vi "Picture Dial.vi"() -> ()   [LabVIEW 2014]
doc: "Combines a picture control with a dial to have a picture within a dial. The picture control is grouped and locked to the dial along with a decoration to cover the corners of the picture control.\n\n*Notice the use of a stored pixmap image so the image is saved with the VI itself."
uses:
  Rotate.llb/rotate 24bit.vi
panel:
  out "new picture":picture
  in  "Duty Cycle %":dbl(slide)=0.05 scale=0.0..180.0
  in  "stop":bool
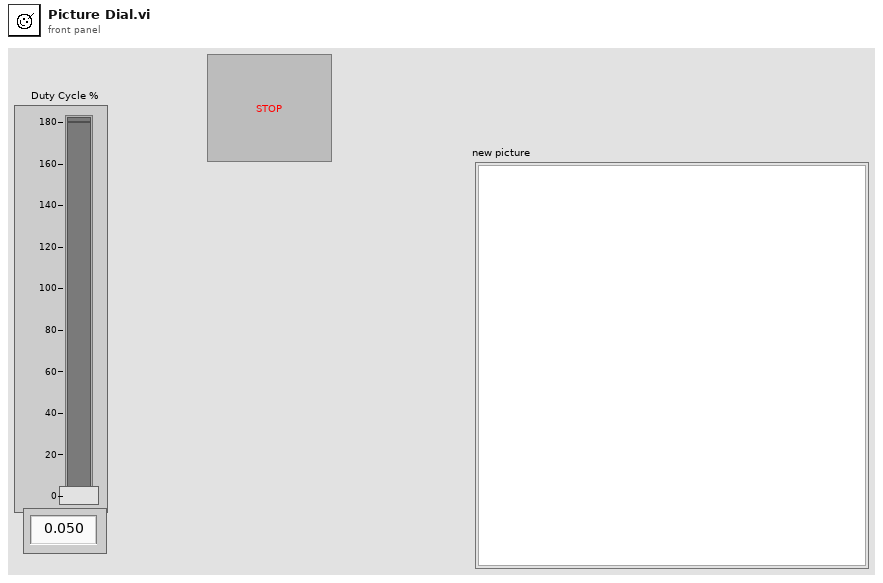
[diagram p1: front panel]
types:
  T1 = typedef "imagedata.ctl" = cluster{"image type":i32, "image depth":i32, "image":u8[], "mask":u8[], "colors":u32[], "Rectangle":cluster{"left":i16, "top":i16, "right":i16, "bottom":i16}}
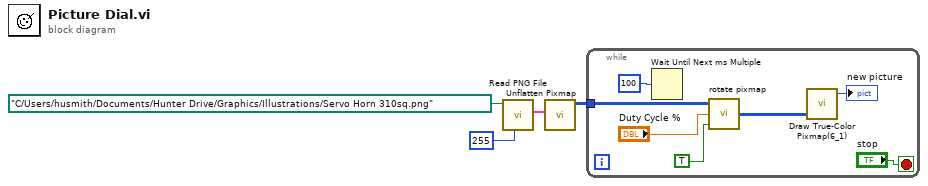
[diagram p0: block diagram]
diagram:
  n1 = call <vilib>:"Read PNG File.vi"("Transparency Thresh"=u8 255, "path to PNG file"=path "C:/Users/husmith/Documents/Hunter Drive/Graphics/Illustrations/Servo Horn 310sq.png") -> ("image data"=w4:T1)  [unwired: 7 in, 2 out]
  n2 = call <vilib>:"Unflatten Pixmap.vi"("image data"=w4) -> ("24-bit pixmap"=w1:u32[][])  [unwired: 4 in, 6 out]
  n3 = while {
    tunnel: w1 -> [w12]
    stop <- "stop" stop-if-true
    n4 = Wait Until Next ms Multiple(millisecond multiple=u32 100) -> ()  [unwired: 1 out]
    n5 = call-poly "rotate pixmap.vi"("Maintain Center Position?"=TRUE, "Rotation Angle (degrees)"="Duty Cycle %", "Pixmap"=w12) -> ("Rotated Pixmap"=w8:u32[][], "Color Table Index of Fill Color"=w5:i32)
    n6 = call <vilib>:"Draw True-Color Pixmap(6_1).vi"("data (RGB format)"=w8) -> ("new picture"=→"new picture":picture)  [unwired: 8 in]
  }
